vi "simple 2.vi"() -> ()   [LabVIEW 2022 SP3]
panel:
  out "Result":dbl
  in  "Number 2":dbl
  in  "Number 1":dbl
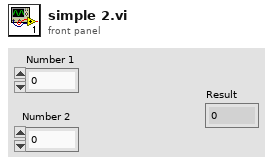
[diagram p1: front panel]
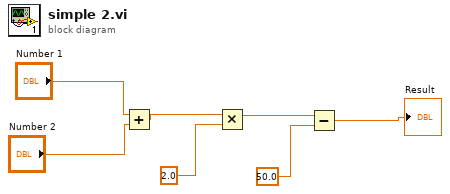
[diagram p0: block diagram]
diagram:
  n1 = Add(x="Number 1", y="Number 2") -> (x+y=w2:dbl)
  n2 = Multiply(x=w2, y=2.0) -> (x*y=w3:dbl)
  n3 = Subtract(x=w3, y=50.0) -> (x-y=→"Result":dbl)
